vi "Write_Settings.vi"(6 "Dialog? (false)":bool, 7 "Options":T8, 8 "Status/Errors in":refnum<vi>, 10 "Control Parameters [] in":T15[](array[typedef]) {"Aux Byte Value" format="%02x"; "Max Real Value" format="%#_6e"; "Min Real Value" format="%#_6e"; "dReal/dByte" format="%#_6e"; "Byte Value" format="%02x"; "Identifier" format="%02x"}, 11 "Main parameters in":T1={"Mode"={"Mode"=enum."Dialog", "Expert?"=FALSE, "Dialog?"=FALSE}, "Stop loop"={"Settings changed?"=FALSE, "Stop?"=refnum}, "Send message"={"Send mode"=enum."Get parameters", "Set parameter list"=0, "Get parameter list"=0, "Reset device"=0, "Length set settings message"=0, "Reset buttons?"=FALSE, "Reset Master?"=enum."General"}, "Write settings"={"Options"=enum."File 1"}, "Settings state"={"MAS locked?"=refnum, "SLV locked?"=refnum}, "Button refs"={"Stop program"=refnum, "Save settings"=refnum, "DAQ mode"=refnum, "Reset settings"=refnum, "Apply settings"=refnum, "Reset MAS"=refnum, "Reset SLV"=refnum, "Local DBase?"=refnum, "Last value DBase"=FALSE, "Database"=refnum, "Calibration"=refnum, "Save settings 2"=refnum}, "Update screen"={"Detector number"=0, "Hardware"=enum."None"}, "Files"={"Path config file"=path "", "Path def. ini file"=path "", "Path ini file 1"=path "", "Path ini file 2"=path "", "Path RBF file"=path ""}, "DB connection"={"connection reference"=refnum, "Connected?"=refnum, "ODBC Name"=""}, "Status_id"=refnum, "Time difference"=refnum, "Satellites"=refnum, "Alignment parameters"=refnum, "Page Statistics 2"=refnum, "Database"=refnum, "Page Statistics"=refnum} {"Update screen"."Detector number" format="%#.0f"; "Send message"."Reset device" format="%x"; "Send message"."Get parameter list" format="%x"; "Send message"."Set parameter list" format="%x"}) -> (0 "Status/Errors out":refnum<vi>, 2 "Control Parameters [] out":T15[](array[typedef]) {"Aux Byte Value" format="%02x"; "Max Real Value" format="%#_6e"; "Min Real Value" format="%#_6e"; "dReal/dByte" format="%#_6e"; "Byte Value" format="%02x"; "Identifier" format="%02x"}, 3 "Main parameters out":T1={"Mode"={"Mode"=enum."Dialog", "Expert?"=FALSE, "Dialog?"=FALSE}, "Stop loop"={"Settings changed?"=FALSE, "Stop?"=refnum}, "Send message"={"Send mode"=enum."Get parameters", "Set parameter list"=0, "Get parameter list"=0, "Reset device"=0, "Length set settings message"=0, "Reset buttons?"=FALSE, "Reset Master?"=enum."General"}, "Write settings"={"Options"=enum."File 1"}, "Settings state"={"MAS locked?"=refnum, "SLV locked?"=refnum}, "Button refs"={"Stop program"=refnum, "Save settings"=refnum, "DAQ mode"=refnum, "Reset settings"=refnum, "Apply settings"=refnum, "Reset MAS"=refnum, "Reset SLV"=refnum, "Local DBase?"=refnum, "Last value DBase"=FALSE, "Database"=refnum, "Calibration"=refnum, "Save settings 2"=refnum}, "Update screen"={"Detector number"=0, "Hardware"=enum."None"}, "Files"={"Path config file"=path "", "Path def. ini file"=path "", "Path ini file 1"=path "", "Path ini file 2"=path "", "Path RBF file"=path ""}, "DB connection"={"connection reference"=refnum, "Connected?"=refnum, "ODBC Name"=""}, "Status_id"=refnum, "Time difference"=refnum, "Satellites"=refnum, "Alignment parameters"=refnum, "Page Statistics 2"=refnum, "Database"=refnum, "Page Statistics"=refnum} {"Update screen"."Detector number" format="%#.0f"; "Send message"."Reset device" format="%x"; "Send message"."Get parameter list" format="%x"; "Send message"."Set parameter list" format="%x"})   [LabVIEW 2010]
uses:
  Controls/Control_Parameters.ctl
  Controls/Master.ctl
  Controls/Write_Settings_Options.ctl
  Controls/Main_Parameters.ctl
  Controls/Mode.ctl
  Controls/Stop_Loop.ctl
  Controls/Send_Message.ctl
  Controls/Send_Message_Mode.ctl
  Controls/Write_Settings.ctl
  Controls/Settings_State.ctl
  Controls/Button_Refs.ctl
  Controls/Update_Screen.ctl
  Controls/Files.ctl
  Controls/DB_Connection.ctl
  database/Connection.llb/Conn ObjectReference.ctl
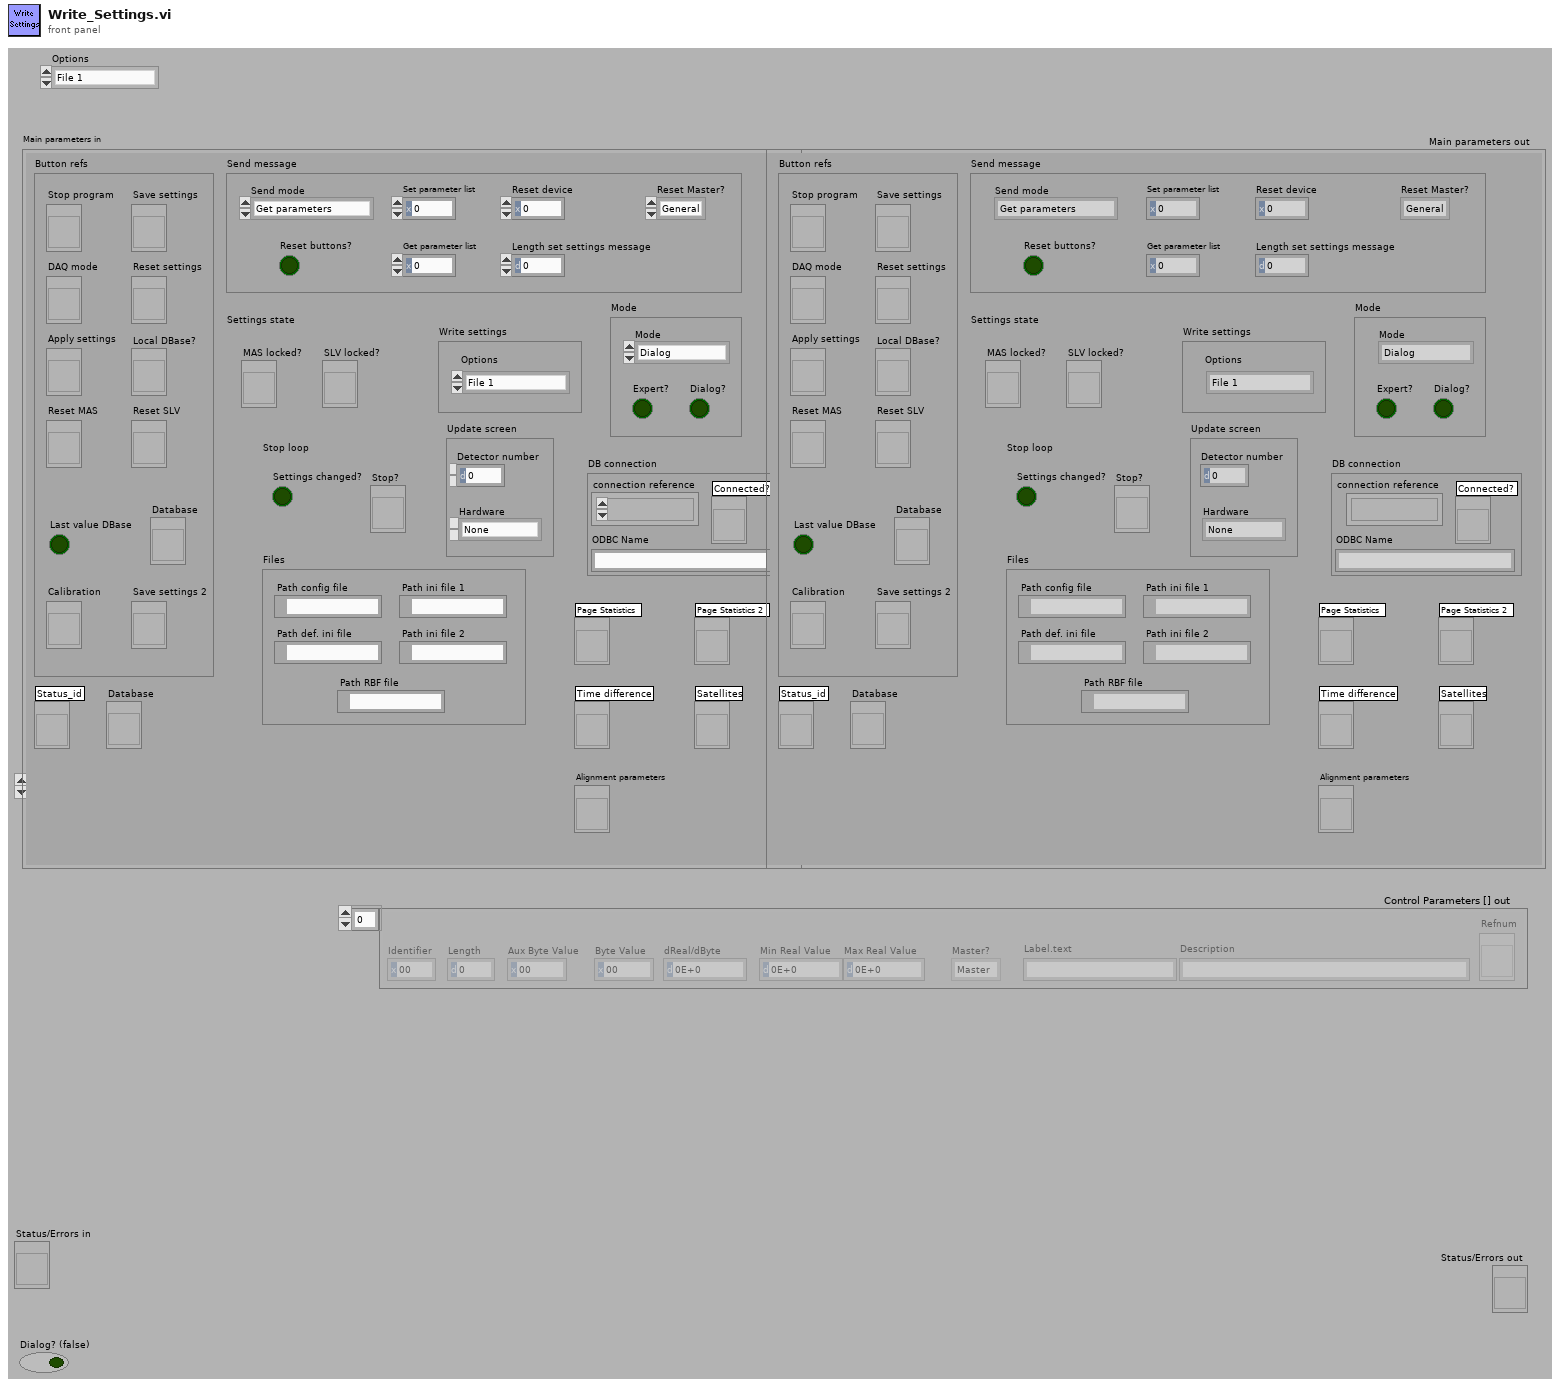
[diagram p1: front panel]
types:
  T1 = typedef "Main_Parameters.ctl" = cluster{"Mode":T2, "Stop loop":T3, "Send message":T4, "Write settings":T7, "Settings state":T9, "Button refs":T10, "Update screen":T11, "Files":T12, "DB connection":T13, "Status_id":refnum<vi>, "Time difference":refnum<vi>, "Satellites":refnum<vi>, "Alignment parameters":refnum<vi>, "Page Statistics 2":refnum<vi>, "Database":refnum<vi>, "Page Statistics":refnum<vi>}
  T2 = typedef "Mode.ctl" = cluster{"Mode":enum8{"Stop", "Dialog", "Hisparc II", "Hisparc II DAQ", "Alignment"}, "Expert?":bool, "Dialog?":bool}
  T3 = typedef "Stop_Loop.ctl" = cluster{"Settings changed?":bool, "Stop?":refnum<vi>}
  T4 = typedef "Send_Message.ctl" = cluster{"Send mode":T5, "Set parameter list":u8, "Get parameter list":u8, "Reset device":u8, "Length set settings message":i32, "Reset buttons?":bool, "Reset Master?":T6}
  T5 = typedef "Send_Message_Mode.ctl" = enum16{"Get parameters", "Set parameters", "From front panel", "From parameters", "Reset device", "Alignment"}
  T6 = typedef "Master.ctl" = enum16{"Master", "Slave", "General"}
  T7 = typedef "Write_Settings.ctl" = cluster{"Options":T8}
  T8 = typedef "Write_Settings_Options.ctl" = enum16{"File 1", "File 2", "Alignment", "Reset"}
  T9 = typedef "Settings_State.ctl" = cluster{"MAS locked?":refnum<vi>, "SLV locked?":refnum<vi>}
  T10 = typedef "Button_Refs.ctl" = cluster{"Stop program":refnum<vi>, "Save settings":refnum<vi>, "DAQ mode":refnum<vi>, "Reset settings":refnum<vi>, "Apply settings":refnum<vi>, "Reset MAS":refnum<vi>, "Reset SLV":refnum<vi>, "Local DBase?":refnum<vi>, "Last value DBase":bool, "Database":refnum<vi>, "Calibration":refnum<vi>, "Save settings 2":refnum<vi>}
  T11 = typedef "Update_Screen.ctl" = cluster{"Detector number":u16, "Hardware":enum8{"None", "HiSPARC I", "HiSPARC II", "HiSPARC III", "Unknown"}}
  T12 = typedef "Files.ctl" = cluster{"Path config file":path, "Path def. ini file":path, "Path ini file 1":path, "Path ini file 2":path, "Path RBF file":path}
  T13 = typedef "DB_Connection.ctl" = cluster{"connection reference":T14, "Connected?":refnum<vi>, "ODBC Name":string}
  T14 = typedef "Conn ObjectReference.ctl" = refnum<k1>
  T15 = typedef "Control_Parameters.ctl" = cluster{"Identifier":u8, "Length":u16, "Byte Value":u32, "dReal/dByte":dbl, "Min Real Value":dbl, "Max Real Value":dbl, "Master?":T6, "Label.text":string, "Description":string, "Refnum":refnum<vi>, "Aux Byte Value":u32}
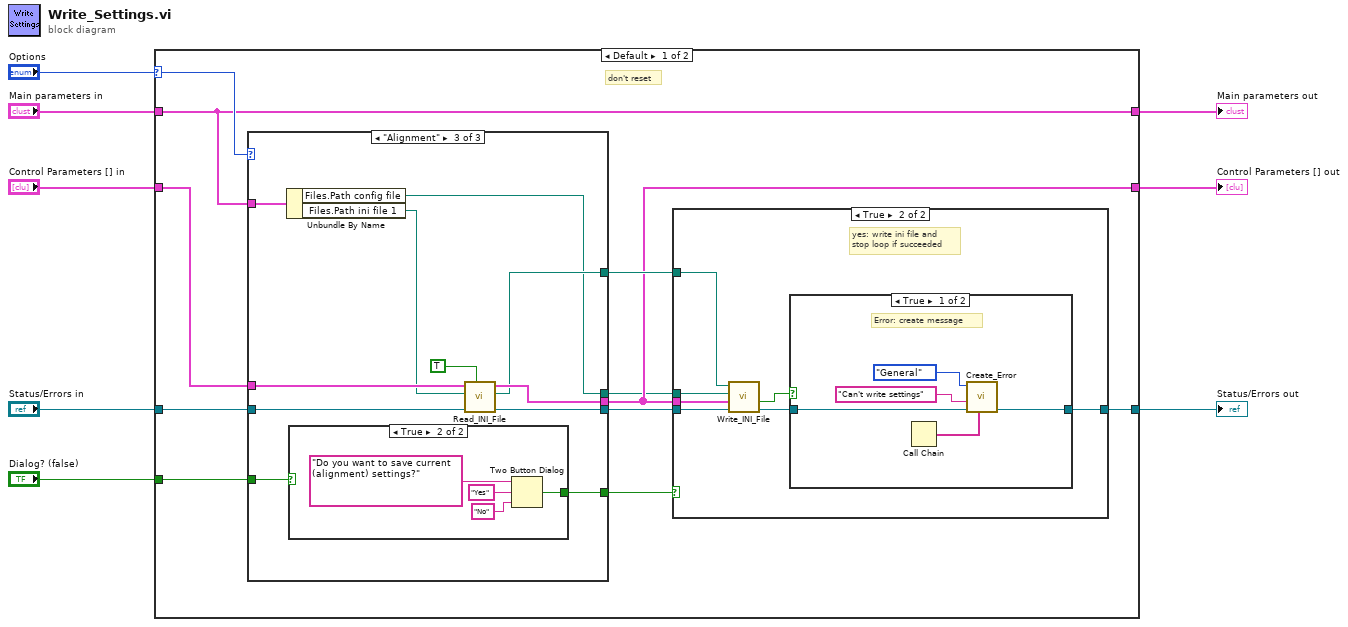
[diagram p0: block diagram]
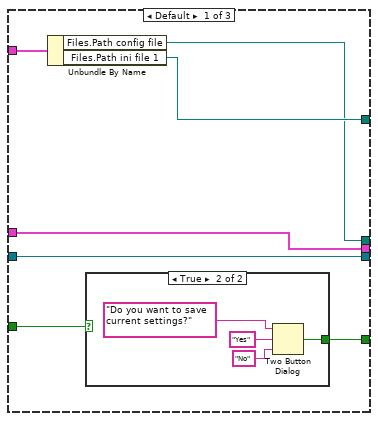
[diagram p2: hidden frame]
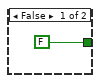
[diagram p3: hidden frame]
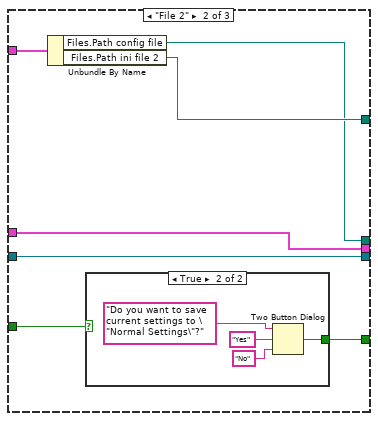
[diagram p4: hidden frame]
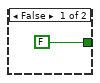
[diagram p5: hidden frame]
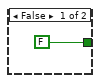
[diagram p6: hidden frame]
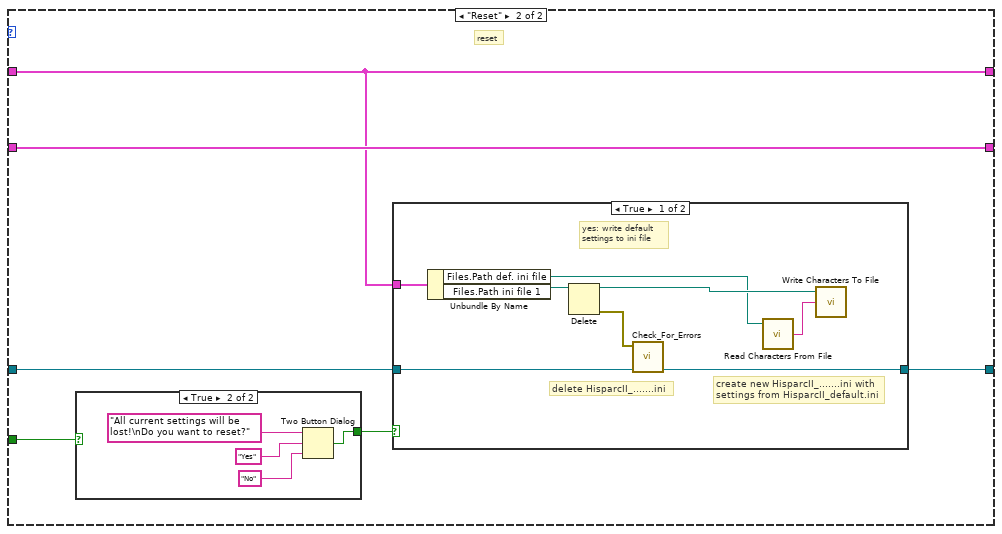
[diagram p9: hidden frame]
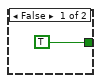
[diagram p11: hidden frame]
diagram:
  n1 = case shown="Default" "Options" {
    selector: "Options" -> [w12 _]
    tunnel: "Dialog? (false)" -> [w19 w79]
    tunnel: [w18 w78] -> w7
    tunnel: "Control Parameters [] in" -> [w14 w76]
    tunnel: "Status/Errors in" -> [w15 w77]
    tunnel: "Main parameters in" -> [w10 w74]
    tunnel: [w10 w74] -> w3
    tunnel: [w13 w76] -> w2
    frame Default {
      # "don't reset"
      n2 = case shown="\"Alignment\"" w12 {
        tunnel: w19 -> [w24 w36 w47]
        tunnel: [w21 w33 w50] -> w17
        tunnel: [w26 w38 w53] -> w16
        tunnel: w15 -> [w26 w38 w54]
        tunnel: [w25 w37 w51] -> w13
        tunnel: w14 -> [w25 w37 w52]
        tunnel: [w23 w35 w48] -> w11
        tunnel: w10 -> [w22 w34 w46]
        tunnel: [w20 w32 w44] -> w9
        frame Default {
          n3 = Unbundle By Name(w22) -> ("Files.Path config file"=w20:path, "Files.Path ini file 1"=w21:path)
          n4 = case shown="True" w24 {
            tunnel: [FALSE ("T button?") w28] -> w23
            frame False {
            }
            frame True {
              n5 = Two Button Dialog(message="Do you want to save current settings?", 1:"No" ("F button name (\"Cancel\")"), 2:"Yes" ("T button name (\"OK\")")) -> (T button?=w28:bool)
            }
          }
        }
        frame "File 2" {
          n6 = Unbundle By Name(w34) -> ("Files.Path config file"=w32:path, "Files.Path ini file 2"=w33:path)
          n7 = case shown="True" w36 {
            tunnel: [FALSE ("T button?") w40] -> w35
            frame False {
            }
            frame True {
              n8 = Two Button Dialog(message="Do you want to save current settings to \"Normal Settings\"?", 1:"No" ("F button name (\"Cancel\")"), 2:"Yes" ("T button name (\"OK\")")) -> (T button?=w40:bool)
            }
          }
        }
        frame "Alignment" {
          n9 = Unbundle By Name(w46) -> ("Files.Path config file"=w44:path, "Files.Path ini file 1"=w45:path)
          n10 = case shown="True" w47 {
            tunnel: [FALSE ("T button?") w56] -> w48
            frame False {
            }
            frame True {
              n11 = Two Button Dialog(message="Do you want to save current (alignment) settings?", 1:"No" ("F button name (\"Cancel\")"), 2:"Yes" ("T button name (\"OK\")")) -> (T button?=w56:bool)
            }
          }
          n12 = call "Read_INI_File.vi"("Calibration mode? (f)"=TRUE, "Status/Errors in"=w54, "Path ini file in"=w45, "Control Parameters [] in"=w52) -> ("Status/Errors out"=w53:refnum<vi>, "Path ini file out"=w50:path, "Control Parameters [] out"=w51:T15[])  [unwired: 5 out]
        }
      }
      n13 = case shown="True" w11 {
        tunnel: w17 -> [_ w67]
        tunnel: w16 -> [w60 w66]
        tunnel: [w60 w64] -> w18
        tunnel: w13 -> [_ w62]
        tunnel: w9 -> [_ w61]
        frame False {
          # "no: don't write ini file\nand stop loop"
        }
        frame True {
          # "yes: write ini file and\nstop loop if succeeded"
          n14 = call "Write_INI_File.vi"("Status/Errors in"=w66, "Control Parameters [] in"=w62, "Path configuration file in"=w61, "Path ini file in"=w67) -> ("Status/Errors out"=w65:refnum<vi>, "Error?"=w63:bool)  [unwired: 6 out]
          n15 = case shown="True" w63 {
            tunnel: w65 -> [w72 w73]
            tunnel: [w71 w73] -> w64
            frame True {
              # "Error: create message"
              n16 = Call Chain() -> (call chain=w68:string[])
              n17 = call "Create_Error.vi"("Call chain"=w68, "Status/Errors in"=w72, "HiSPARC error"="Can't write settings", "Master?"=Master."General") -> ("Status/Errors out"=w71:refnum<vi>)  [unwired: 2 in, 5 out]
            }
            frame False {
              # "no error"
            }
          }
        }
      }
    }
    frame "Reset" {
      # "reset"
      n18 = case shown="True" w79 {
        tunnel: [TRUE ("T button?") w93] -> w75
        frame False {
        }
        frame True {
          n19 = Two Button Dialog(message="All current settings will be lost!\nDo you want to reset?", 1:"No" ("F button name (\"Cancel\")"), 2:"Yes" ("T button name (\"OK\")")) -> (T button?=w93:bool)
        }
      }
      n20 = case shown="True" w75 {
        tunnel: w77 -> [w84 w88]
        tunnel: [w83 w88] -> w78
        tunnel: w74 -> [w82 _]
        frame True {
          # "create new HisparcII_.......ini with\nsettings from HisparcII_default.ini"
          # "delete HisparcII_.......ini"
          # "yes: write default\nsettings to ini file"
          n21 = Unbundle By Name(w82) -> ("Files.Path def. ini file"=w80:path, "Files.Path ini file 1"=w81:path)
          n22 = Delete(path (use dialog)=w81) -> (deleted path=w86:path, error out=w87:errorcluster)  [unwired: 1 in, 4 out]
          n23 = call "Check_For_Errors.vi"("Status/Errors in"=w84, "error in"=w87) -> ("Status/Errors out"=w83:refnum<vi>)  [unwired: 9 out]
          n24 = call <vilib>:"Read Characters From File.vi"("file path (dialog if empty)"=w80) -> ("character string"=w85:string)  [unwired: 1 in, 7 out]
          n25 = call <vilib>:"Write Characters To File.vi"("character string"=w85, "file path (dialog if empty)"=w86) -> ()  [unwired: 1 in, 3 out]
        }
        frame False {
          # "no: don't write default\nsettings to ini file"
        }
      }
    }
  }
  "Control Parameters [] out" <- w2
  "Status/Errors out" <- w7
  "Main parameters out" <- w3
